vi "UnexpectedDepsCheck1.vi"(6 "StatusIndicator Ref":refnum<vi>, 8 "error in (no error)":errorcluster, 10 "LibraryNames":string[](array[string]), 11 "Workspace Path":path=path "E:/sw-deps-monitor") -> (0 "error out":errorcluster)   [LabVIEW 2023, in "CICD.lvlib"]
uses:
  CICD.lvlib
  <vilib>/Utility/config.llb/NI_LVConfig.lvlib
  Typedefs/DepsCheckResult.ctl
panel:
  out "Failures":T1[](array[typedef])
  out "Status Indicator":string
  # "Leave Empty to check all Libraries"
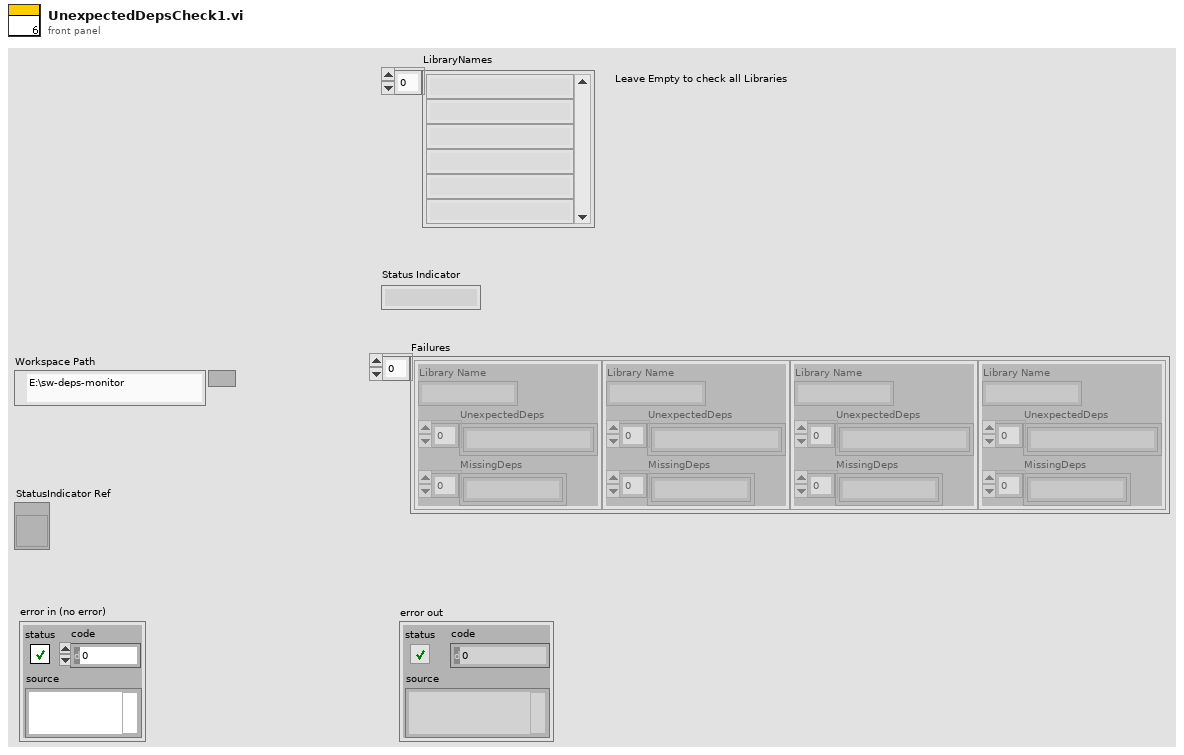
[diagram p1: front panel]
types:
  T1 = typedef "CICD.lvlib/DepsCheckResult.ctl" = cluster{"Library Name":string, "UnexpectedDeps":string[], "MissingDeps":string[]}
  T2 = typedef "NI_LVConfig.lvlib/Config Data RefNum.ctl" = refnum<k1>
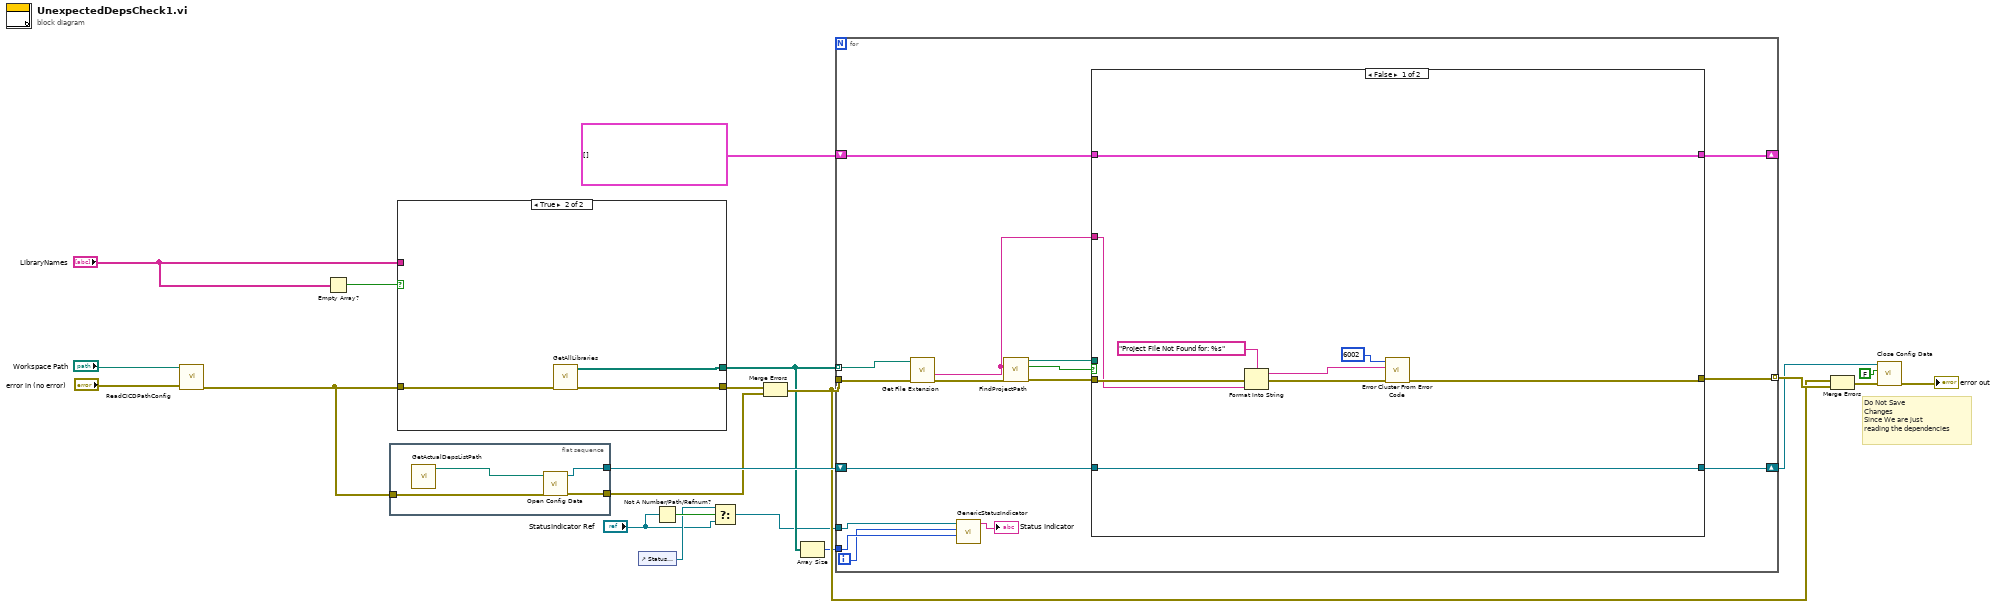
[diagram p0: block diagram]
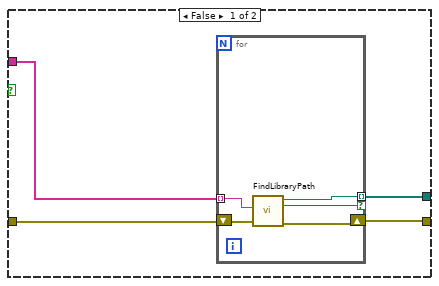
[diagram p2: hidden frame]
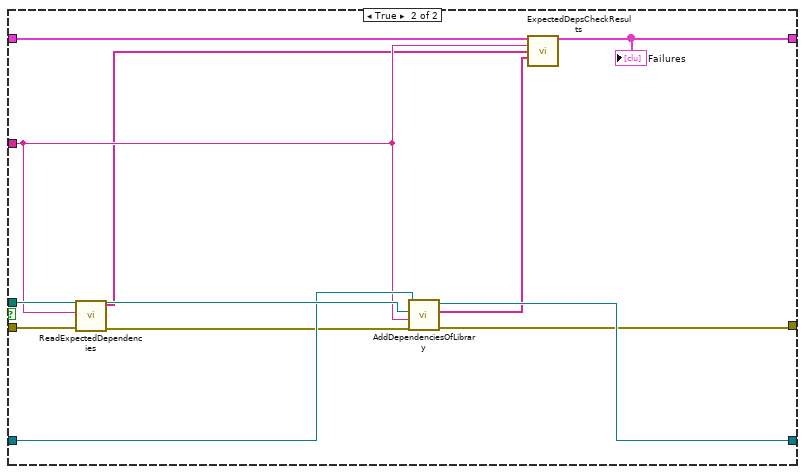
[diagram p3: hidden frame]
diagram:
  # "Do Not Save\nChanges\nSince We are just\nreading the dependencies"
  n1 = call "ReadCICDPathConfig.vi"("error in (no error)"="error in (no error)", "Workspace Path"="Workspace Path") -> ("error out"=w1:errorcluster)  [unwired: 8 in, 1 out]
  n2 = Empty Array?(array="LibraryNames") -> (empty?=w14:bool)
  n3 = flat-sequence {
    tunnel: [w25] -> w20
    tunnel: [w24] -> w16
    tunnel: w1 -> [w22]
    frame #0 {
      n4 = call "GetActualDepsListPath.vi"() -> ("Path"=w23:path)  [unwired: 11 in]
      n5 = call <vilib>:"Open Config Data.vi"("error in (no error)"=w22, "configuration file path"=w23) -> ("error out"=w24:errorcluster, "refnum"=w25:T2)  [unwired: 7 in, 1 out]
    }
  }
  n6 = case shown="True" w14 {
    tunnel: w1 -> [w29 w35]
    tunnel: [w27 w37] -> w11
    tunnel: "LibraryNames" -> [w28 _]
    tunnel: [w26 w36] -> w12
    frame False {
      n7 = for {
        tunnel: w28 -> [w33] mode=indexing
        shift-right: [w32] -> w26
        shift-left: w29 -> [w34]
        tunnel: [w31] -> w27 mode=indexing if=w30
        n8 = call "FindLibraryPath.vi"("error in (no error)"=w34, "Library Name"=w33) -> ("error out"=w32:errorcluster, "Found?"=w30:bool, "Library Path"=w31:path)  [unwired: 7 in]
      }
    }
    frame True {
      n9 = call "GetAllLibraries.vi"("error in (no error)"=w35) -> ("error out"=w36:errorcluster, "Lvlib paths"=w37:path[])  [unwired: 9 in]
    }
  }
  n10 = control-ref of="Status Indicator"() -> (w8:refnum<vi>)
  n11 = Not A Number/Path/Refnum?(number/path/refnum="StatusIndicator Ref") -> (NaN/Path/Refnum?=w9:bool)
  n12 = Select(t=w8, s=w9, f="StatusIndicator Ref") -> (s? t:f=w6:refnum<vi>)
  n13 = Merge Errors(w12, w16) -> (w15:errorcluster)
  n14 = Array Size(array=w11) -> (size(s)=w10:i32)
  n15 = for {
    tunnel: w15 -> [w53]
    tunnel: w11 -> [w51] mode=indexing
    tunnel: [w52] -> w21 mode=indexing
    shift-right: [w45] -> w17
    shift-left: w20 -> [w46]
    tunnel: w6 -> [w43]
    tunnel: w10 -> [w42]
    shift-right: [w38] -> _
    shift-left: T1[] [] -> [w39]
    i -> [w41]
    n16 = call <vilib>:"Get File Extension.vi"("error in (no error)"=w53, "file"=w51) -> ("error out"=w50:errorcluster, "filename without extension"=w44:string)  [unwired: 5 in, 3 out]
    n17 = call "GenericStatusIndicator.vi"("Total"=w42, "Current Iteration"=w41, "String in"=w43) -> ("Status"=→"Status Indicator":string)  [unwired: 8 in]
    n18 = call "FindProjectPath.vi"("error in (no error)"=w50, "Library Name"=w44) -> ("error out"=w48:errorcluster, "Found?"=w49:bool, "Project Path"=w47:path)  [unwired: 7 in]
    n19 = case shown="False" w49 {
      tunnel: w48 -> [w58 w70]
      tunnel: [w60 w68] -> w52
      tunnel: w47 -> [_ w73]
      tunnel: w46 -> [w62 w72]
      tunnel: [w62 w71] -> w45
      tunnel: w44 -> [w56 w66]
      tunnel: w39 -> [w61 w67]
      tunnel: [w61 w63] -> w38
      frame False {
        n20 = Format Into String(format string="Project File Not Found for: %s", error in=w58, w56) -> (resulting string=w55:string, error out=w54:errorcluster)  [unwired: 1 in]
        n21 = call <vilib>:"Error Cluster From Error Code.vi"("error in (no error)"=w54, "error message (\"\")"=w55, "error code (0)"=6002) -> ("error out"=w60:errorcluster)  [unwired: 6 in]
      }
      frame True {
        n22 = call "ReadExpectedDependencies.vi"("error in (no error)"=w70, "Library Name"=w66) -> ("error out"=w69:errorcluster, "ExpectedDependencies"=w65:string[])  [unwired: 6 in, 2 out]
        n23 = call "AddDependenciesOfLibrary.vi"("error in (no error)"=w69, "LibraryName"=w66, "Project Path"=w73, "Config Refnum in"=w72) -> ("error out"=w68:errorcluster, "ActualDependencies"=w64:string[], "Config Refnum out"=w71:T2)  [unwired: 5 in]
        n24 = call "ExpectedDepsCheckResults.vi"("ResultsArray"=w67, "Library Name"=w66, "ExpectedDependencies"=w65, "ActualDependencies"=w64) -> ("ResultsArray out"=w63:T1[])  [unwired: 11 in]
        "Failures" <- w63
      }
    }
  }
  n25 = Merge Errors(w15, w21) -> (w19:errorcluster)
  n26 = call <vilib>:"Close Config Data.vi"("error in (no error)"=w19, "write file if changed (T)"=FALSE, "refnum"=w17) -> ("error out"=→"error out":errorcluster)  [unwired: 7 in, 1 out]
